vi "WriteFile.vi"(8 "error in (no error)":errorcluster, 11 "Excel refnum":T1) -> (0 "error out":errorcluster, 3 "Excel refnum out":T1)   [LabVIEW 2020, in "NI_ExcelFile.lvlib"]
doc: "Writes data that you logged with the WriteData VI to the specified .xlsx file. After you finish the writing operation, use the Destroy VI to close the reference of the .xlsx file and to delete temporary files.\n \nExcel refnum: Specifies a reference to the .xlsx file on which to perform the operation. Use the Create VI to create or open the refnum.\n\nerror in: describes error conditions that occur before this node runs. This input provides standard error in functionality.\n\nExcel refnum out: Returns a Microsoft Excel file reference to the .xlsx file on which you performed the operation.\n\nerror out: contains error information. This output provides standard error out functionality."
uses:
  <vilib>/express/express shared/NI_ExcelFile/NI_ExcelFile.lvlib
  <vilib>/express/express shared/NI_ExcelFile/Ctrls/ExcelRefnum.ctl
  <vilib>/express/express shared/NI_ExcelFile/Ctrls/MainData.ctl
  <vilib>/express/express shared/NI_ExcelFile/Ctrls/StreamMode.ctl
  <vilib>/express/express shared/NI_ExcelFile/Ctrls/TimeColumnMode.ctl
  <vilib>/express/express shared/NI_ExcelFile/Ctrls/FileAttribute.ctl
  <vilib>/express/express shared/NI_ExcelFile/Ctrls/Columns.ctl
  <vilib>/express/express shared/NI_ExcelFile/Ctrls/ColumnInfo.ctl
  <vilib>/express/express shared/NI_ExcelFile/Ctrls/DataType.ctl
  <vilib>/express/express shared/NI_ExcelFile/Ctrls/wd_recordInfo.ctl
  <vilib>/express/express shared/NI_ExcelFile/Ctrls/disk_TemplateFile.ctl
  <vilib>/express/express shared/NI_ExcelFile/Ctrls/meta_file.ctl
  <vilib>/express/express shared/NI_ExcelFile/Ctrls/meta_Block.ctl
  <vilib>/express/express shared/NI_ExcelFile/Ctrls/meta_BlockType.ctl
  <vilib>/express/express shared/NI_ExcelFile/Ctrls/meta_FileInfo.ctl
  <vilib>/express/express shared/NI_ExcelFile/Ctrls/meta_FileInfo_2013.ctl
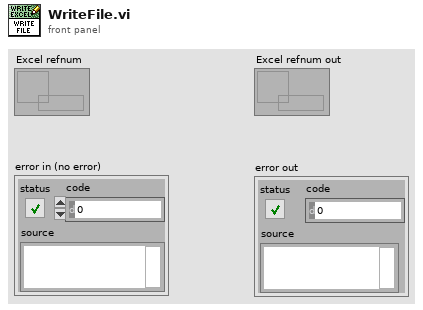
[diagram p1: front panel]
types:
  T1 = typedef "NI_ExcelFile.lvlib/ExcelRefnum.ctl" = refnum<data-value>
  T2 = typedef "NI_ExcelFile.lvlib/meta_FileInfo_2013.ctl" = cluster{"NextPosition":i64, "NextRow":i32, "FileAttribute ":T3}
  T3 = typedef "NI_ExcelFile.lvlib/FileAttribute.ctl" = cluster{"Creator":string, "Title":string, "SheetName":string}
  T4 = typedef "NI_ExcelFile.lvlib/meta_FileInfo.ctl" = cluster{"meta_FileInfo_2013":T2}
  T5 = typedef "NI_ExcelFile.lvlib/MainData.ctl" = cluster{"TargetFile":path, "StreamMode":T6, "Append?":bool, "ChunkSize":u64, "TimeColumnMode":T7, "TimestampFormat":string, "AbsoluteTime?":bool, "FileAttribute ":T3, "Column":T8, "FileRef":refnum<k1>, "MemoryRef":refnum<data-value>[], "RecordInfo":T11[], " ChannelPreviousInfo":u32[], "ChannelFirstRecord":u32[], "PredefinedFormattedValueLength":i64, "DiskTemplate":T12}
  T6 = typedef "NI_ExcelFile.lvlib/StreamMode.ctl" = enum16{"File", "Memory"}
  T7 = typedef "NI_ExcelFile.lvlib/TimeColumnMode.ctl" = enum16{"Empty", "OnePerCh", "One"}
  T8 = typedef "NI_ExcelFile.lvlib/Columns.ctl" = T9[]
  T9 = typedef "NI_ExcelFile.lvlib/ColumnInfo.ctl" = cluster{"Header":string, "Format":string, "DataType":T10, "Length":u64}
  T10 = typedef "NI_ExcelFile.lvlib/DataType.ctl" = enum16{"DDT", "WFM", "Array of STR", "Array of DBL", "Array of I8", "Array of I16", "Array of I32", "Array of I64", "Array of SGL", "Array of U8", "Array of U16", "Array of U32", "Array of U64", "Array of Time"}
  T11 = typedef "NI_ExcelFile.lvlib/wd_recordInfo.ctl" = cluster{"ChannelIndex":u32, "StartIndex":u64, "Length":u64, "Previous":i32, "Next":i32}
  T12 = typedef "NI_ExcelFile.lvlib/disk_TemplateFile.ctl" = cluster{"XMLRef":refnum<file>[], "ZipPath":path, "MetaFile":T13, "TempFolder":path}
  T13 = typedef "NI_ExcelFile.lvlib/meta_file.ctl" = cluster{"Ref":refnum<file>, "NextRow":i32, "NextPosition":i64, "Block":T14[]}
  T14 = typedef "NI_ExcelFile.lvlib/meta_Block.ctl" = cluster{"Version":u16, "Type":T15, "Length":i32, "Data":string}
  T15 = typedef "NI_ExcelFile.lvlib/meta_BlockType.ctl" = enum16{"NITag", "File", "Column"}
  T16 = typedef "NI_ExcelFile.lvlib/fmt_formatBuffer.ctl" = cluster{"FormatBuffer":u8[], "BufferIndices":i32[], "CellFormatBuffer":u8[], "FormatBufferWidth":i32, "FormattedDataLength":i32, "MaxRow":i32, "StartRow":i32, "TimeColumnMode":T7, "StartTime":timestamp, "Columns":T8, "ActualLength":i32}
  T17 = typedef "NI_ExcelFile.lvlib/data_AllTypeData.ctl" = cluster{"DataType":T10, "DBL":dbl[], "WFM":waveform(dbl), "STR":string[], "Time":timestamp[], "I8":i8[], "I16":i16[], "I32":i32[], "I64":i64[], "SGL":sgl[], "U8":u8[], "U16":u16[], "U32":u32[], "U64":u64[]}
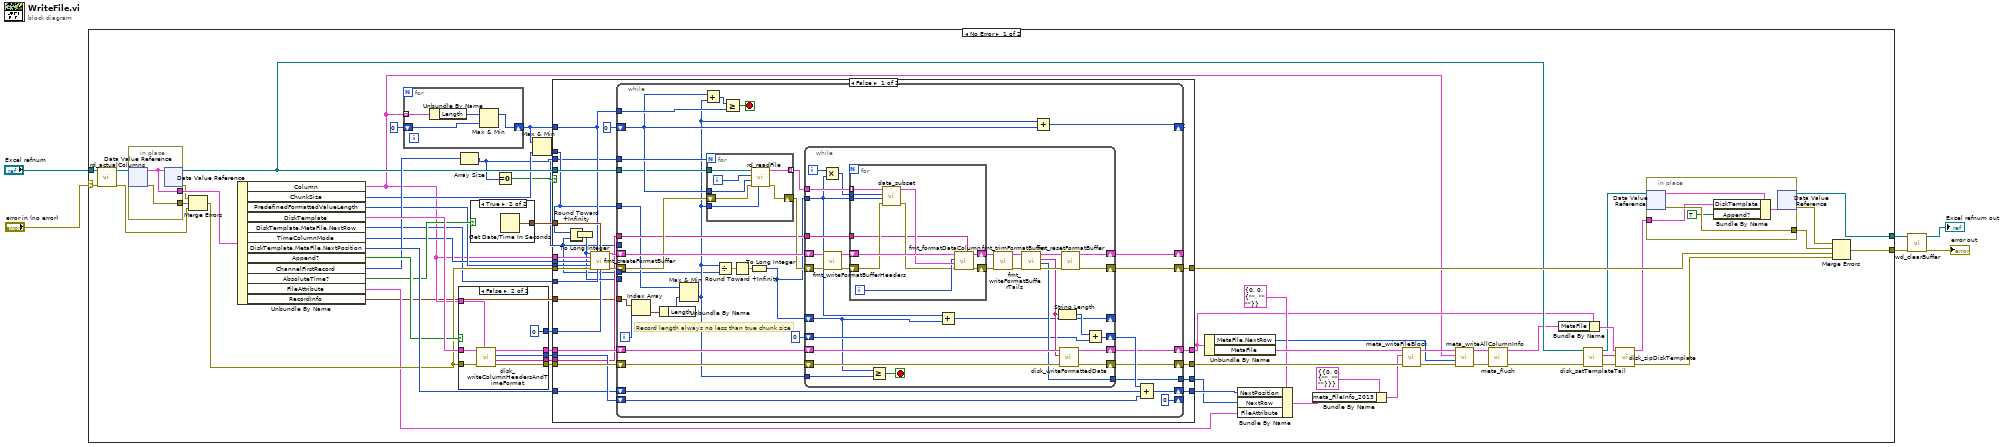
[diagram p0: block diagram]
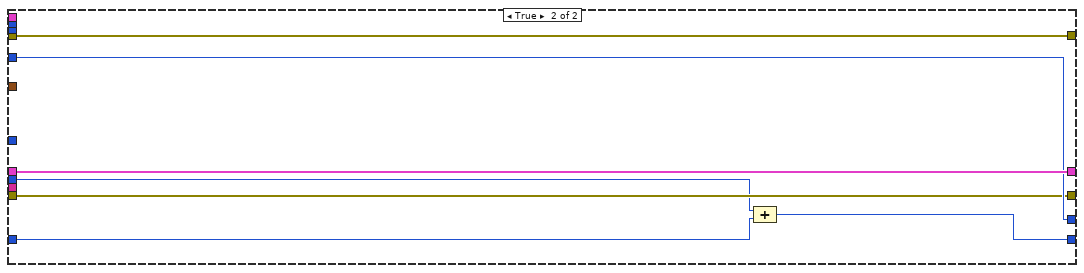
[diagram p2: hidden frame]
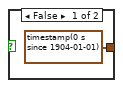
[diagram p3: hidden frame]
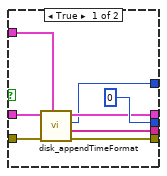
[diagram p4: hidden frame]
diagram:
  n1 = case shown="No Error" "error in (no error)" {
    selector: "error in (no error)" -> [w46 w214]
    tunnel: "Excel refnum" -> [w47 w213]
    tunnel: [w27 w214] -> w2
    tunnel: [w28 w213] -> w4
    frame No Error {
      n2 = call <vilib>:"rd_actualColumns.vi"("error in (no error)"=w46, "Excel refnum"=w47) -> ("errorout"=w45:errorcluster, "Excel refnum out"=w44:T1)  [unwired: 8 in]
      n3 = in-place {
        in-place-border: [w212] -> w60
        in-place-border: [w211] -> w58
        n4 = in-place-dvr #1(w44) -> (w212:T5, w211:errorcluster)
        n5 = in-place-dvr #1(w212) -> (w32:T1, w59:errorcluster)
      }
      n6 = Merge Errors(w59, w58, w45) -> (w43:errorcluster)
      n7 = Unbundle By Name(w60) -> ("Column"=w9:T8, "ChunkSize"=w22:u64, "PredefinedFormattedValueLength"=w26:i64, "DiskTemplate"=w64:T12, "DiskTemplate.MetaFile.NextRow"=w24:i32, "TimeColumnMode"=w25:T7, "DiskTemplate.MetaFile.NextPosition"=w53:i64, "Append?"=w50:bool, "ChannelFirstRecord"=w42:u32[], "AbsoluteTime?"=w41:bool, "FileAttribute"=w13:T3, "RecordInfo"=w7:T11[])
      n8 = for {
        tunnel: w9 -> [w189] mode=indexing
        shift-right: [w188] -> w23
        shift-left: u64 0 ("Column Length") -> [w186]
        n9 = Unbundle By Name(w189) -> ("Length"=w187:u64)
        n10 = Max & Min(x=w187, y=w186) -> (max(x,y)=w188:u64)  [unwired: 1 out]
      }
      n11 = case shown="False" w50 {
        tunnel: w64 -> [w192 w205]
        tunnel: [w191 w204] -> w63
        tunnel: [w195 w203] -> w62
        tunnel: [0 ("formatted header length") w202] -> w61
        tunnel: w43 -> [w196 w199]
        tunnel: [w194 w201] -> w48
        tunnel: w9 -> [w193 w200]
        tunnel: [w190 0 ("max existed styles")] -> w8
        frame True {
          n12 = call <vilib>:"disk_appendTimeFormat.vi"("columns"=w193, "error in (no error)"=w196, "DiskTemplate"=w192) -> ("error out"=w195:errorcluster, "styles map"=w194:string[], "max existed styles"=w190:i32, "DiskTemplate out"=w191:T12)  [unwired: 5 in]
        }
        frame False {
          n13 = call <vilib>:"disk_writeColumnHeadersAndTimeFormat.vi"("column"=w200, "error in"=w199, "DiskTemplate in"=w205) -> ("error out"=w203:errorcluster, "styles map"=w201:string[], "formatted header length"=w202:i32, "DiskTemplate out"=w204:T12)  [unwired: 5 in]
        }
      }
      n14 = Array Size(array=w42) -> (size(s)=w12:i32)
      n15 = case shown="True" w41 {
        tunnel: [timestamp(0 s since 1904-01-01) ("start time") w185] -> w40
        frame False {
        }
        frame True {
          n16 = Get Date/Time In Seconds() -> (seconds since 1Jan1904=w185:timestamp)
        }
      }
      n17 = Equal To 0?(x=w12) -> (x = 0?=w11:bool)
      n18 = Max & Min(x=w23, y=w22) -> (min(x,y)=w14:u64)  [unwired: 1 out]
      n19 = case shown="False" w11 {
        tunnel: [w93 w180] -> w65
        tunnel: w63 -> [w89 w183]
        tunnel: w62 -> [w88 w181]
        tunnel: w61 -> [w87 w179]
        tunnel: w53 -> [w86 w178]
        tunnel: [w84 w181] -> w52
        tunnel: w48 -> [w83 _]
        tunnel: w43 -> [w82 w180]
        tunnel: w40 -> [w81 _]
        tunnel: [w80 w177] -> w34
        tunnel: [w79 w182] -> w33
        tunnel: w32 -> [w78 _]
        tunnel: w26 -> [w77 _]
        tunnel: w25 -> [w76 _]
        tunnel: w24 -> [w75 w182]
        tunnel: w23 -> [w74 _]
        tunnel: w14 -> [w73 _]
        tunnel: w9 -> [w72 _]
        tunnel: w12 -> [w66 _]
        tunnel: [w85 w183] -> w10
        tunnel: w8 -> [w68 _]
        tunnel: w7 -> [w67 _]
        frame False {
          n20 = Divide(x=w73, y=w66) -> (x/y=w70:dbl)
          n21 = Round Toward +Infinity(x=w70) -> (ceil(x): smallest int >= x=w69:dbl)
          n22 = To Long Integer(number=w69) -> (32bit integer=w71:i32)
          n23 = call <vilib>:"fmt_createFormatBuffer.vi"("rows"=w71, "max rows"=w74, "start time"=w81, "columns"=w72, "time column mode"=w76, "predifed formatted value length"=w77, "error in (no error)"=w82, "start row"=w75, "max styles"=w68) -> ("Format buffers out"=w90:T16, "error out"=w91:errorcluster)  [unwired: 5 in]
          n24 = while {
            tunnel: w66 -> [w128]
            tunnel: w74 -> [w127]
            shift-right: [w124] -> w93
            shift-left: w91 -> [w108]
            shift-right: [w114] -> w85
            shift-left: w89 -> [w117]
            shift-right: [w123] -> _
            shift-left: u64 0 ("Trunck size") -> [w120]
            shift-right: [w122] -> _
            shift-left: w90 -> [w125]
            tunnel: w73 -> [w100]
            tunnel: w78 -> [w119]
            shift-right: [w115] -> w84
            shift-left: w88 -> [w118]
            shift-right: [w113] -> w80
            shift-left: w86 -> [w112]
            tunnel: [w110] -> w79
            tunnel: w83 -> [w106]
            shift-right: [0 ("formatted header length")] -> _
            shift-left: w87 -> [w111]
            tunnel: w66 -> [_]
            tunnel: w71 -> [_]
            tunnel: w67 -> [w103]
            tunnel: w66 -> [w96]
            i -> [w102]
            stop <- w126 stop-if-true
            # "Record length always no less than true chunk size"
            n25 = Index Array(array=w103, index=w102) -> (element=w101:T11)
            n26 = Unbundle By Name(w101) -> ("Length"=w94:u64)
            n27 = Max & Min(x=w100, y=w94) -> (min(x,y)=w97:u64)  [unwired: 1 out]
            n28 = Add(x=w120, y=w97) -> (x+y=w121:u64)
            n29 = for {
              N: w128 -> [_]
              tunnel: w97 -> [w175]
              tunnel: w120 -> [w176]
              tunnel: w119 -> [w174]
              shift-right: [w171] -> w107
              shift-left: w108 -> [w172]
              tunnel: [w170] -> w105 mode=indexing
              i -> [w173]
              n30 = call <vilib>:"rd_readFile.vi"("length"=w175, "error in (no error)"=w172, "start index"=w176, "channel index"=w173, "Excel refumn"=w174) -> ("error out"=w171:errorcluster, "data_AllTypeData"=w170:T17)  [unwired: 5 in]
            }
            n31 = Divide(x=w97, y=w96) -> (x/y=w99:dbl)
            n32 = Greater Or Equal?(x=w121, y=w127) -> (x >= y?=w126:bool)
            n33 = Round Toward +Infinity(x=w99) -> (ceil(x): smallest int >= x=w98:dbl)
            n34 = To Long Integer(number=w98) -> (32bit integer=w95:i32)
            n35 = while {
              tunnel: [w145] -> w110
              shift-right: [w152] -> w122
              shift-left: w125 -> [w158]
              shift-right: [w153] -> w124
              shift-left: w107 -> [w154]
              shift-right: [w147] -> w115
              shift-left: w118 -> [w150]
              shift-right: [w146] -> w114
              shift-left: w117 -> [w149]
              shift-right: [w140] -> w116
              shift-left: 0 -> [w139]
              tunnel: w105 -> [w137]
              tunnel: w106 -> [w136]
              tunnel: w95 -> [w130]
              shift-right: [w133] -> _
              shift-left: w95 -> [w129]
              tunnel: w97 -> [w132]
              i -> [w135]
              stop <- w131 stop-if-true
              n36 = Multiply(x=w135, y=w130) -> (x*y=w134:i32)
              n37 = call <vilib>:"fmt_writeFormatBufferHeaders.vi"("error in (no error)"=w154, "Format buffers in"=w158) -> ("error out"=w141:errorcluster, "Format buffers out"=w142:T16)  [unwired: 8 in]
              n38 = for {
                shift-right: [w168] -> w143
                shift-left: w142 -> [w167]
                shift-right: [w169] -> w144
                shift-left: w141 -> [w162]
                tunnel: w137 -> [w166] mode=indexing
                tunnel: w136 -> [w161]
                tunnel: w134 -> [w160]
                tunnel: w130 -> [w159]
                i -> [w164]
                n39 = call <vilib>:"data_subset.vi"("error in (no error)"=w162, "length"=w159, "index"=w160, "data"=w166) -> ("error out"=w163:errorcluster, "data subset"=w165:T17)  [unwired: 6 in]
                n40 = call <vilib>:"fmt_formatDataColumn.vi"("styles map"=w161, "error in (no error)"=w163, "data"=w165, "channel index"=w164, "Format buffers in"=w167) -> ("error out"=w169:errorcluster, "Format buffers out"=w168:T16)  [unwired: 5 in]
              }
              n41 = Greater Or Equal?(x=w129, y=w132) -> (x >= y?=w131:bool)
              n42 = Add(x=w130, y=w129) -> (x+y=w133:i32)
              n43 = call <vilib>:"fmt_writeFormatBufferTails.vi"("error in (no error)"=w144, "Format buffers in"=w143) -> ("error out"=w156:errorcluster, "Format buffers out"=w157:T16)  [unwired: 8 in]
              n44 = call <vilib>:"fmt_trimFormatBuffer.vi"("error in (no error)"=w156, "format buffers in"=w157) -> ("error out"=w151:errorcluster, "max row"=w145:i32, "xml"=w148:string, "format buffers out"=w155:T16)  [unwired: 6 in]
              n45 = String Length(string=w148) -> (length=w138:i32)
              n46 = call <vilib>:"disk_writeFormattedData.vi"("error in"=w150, "xml"=w148, "DiskTemplate in"=w149) -> ("error out"=w147:errorcluster, "DiskTemplate out"=w146:T12)  [unwired: 7 in]
              n47 = call <vilib>:"fmt_resetFormatBuffer.vi"("error in (no error)"=w151, "Format buffers in"=w155) -> ("error out"=w153:errorcluster, "Format buffers out"=w152:T16)  [unwired: 8 in]
              n48 = Add(x=w138, y=w139) -> (x+y=w140:i32)
            }
            n49 = Add(x=w97, y=w120) -> (x+y=w123:u64)
            n50 = Compound Arithmetic op=ADD(w116, w112, w111) -> (w113:i64)
          }
        }
        frame True {
          n51 = Compound Arithmetic op=ADD(w179, w178) -> (w177:i64)
        }
      }
      n52 = Unbundle By Name(w10) -> ("MetaFile.NextRow"=w15:i32, "MetaFile"=w39:T13)
      n53 = Bundle By Name(cluster=T2 {"NextPosition"=0, "NextRow"=0, "FileAttribute "={"Creator"="", "Title"="", "SheetName"=""}} ("meta_FileInfo_2013"), "NextPosition"=w34, "NextRow"=w33, "FileAttribute"=w13) -> (w36:T2)
      n54 = Bundle By Name(cluster=T4 {"meta_FileInfo_2013"={"NextPosition"=0, "NextRow"=0, "FileAttribute "={"Creator"="", "Title"="", "SheetName"=""}}} ("meta_FileInfo"), "meta_FileInfo_2013"=w36) -> (w37:T4)
      n55 = call <vilib>:"meta_writeFileBlock.vi"("error in (no error)"=w52, "meta_FileInfo"=w37, "meta file in"=w39) -> ("error out"=w21:errorcluster, "meta file out"=w20:T13)  [unwired: 7 in]
      n56 = call <vilib>:"meta_writeAllColumnInfo.vi"("error in (no error)"=w21, "start row"=w15, "Column"=w9, "meta file in"=w20) -> ("error out"=w19:errorcluster, "meta file out"=w16:T13)  [unwired: 6 in]
      n57 = call <vilib>:"meta_flush.vi"("error in (no error)"=w19, "meta file in"=w16) -> ("error out"=w18:errorcluster, "meta file out"=w17:T13)  [unwired: 8 in]
      n58 = Bundle By Name(cluster=w10, "MetaFile"=w17) -> (w51:T12)
      n59 = call <vilib>:"disk_setTemplateTail.vi"("error in (no error)"=w18, "Excel refnum"=w32) -> ("error out"=w31:errorcluster, "template tail"=w30:string[], "Excel refnum out"=w29:T1)  [unwired: 7 in]
      n60 = call <vilib>:"disk_zipDiskTemplate.vi"("error in (no error)"=w31, "template tail"=w30, "DiskTemplate in"=w51) -> ("error out"=w54:errorcluster, "DiskTemplate out"=w55:T12)  [unwired: 7 in]
      n61 = in-place {
        in-place-border: [w210] -> w56
        in-place-border: w55 -> [w207]
        n62 = in-place-dvr #2(w29) -> (w209:T5, w210:errorcluster)
        n63 = Bundle By Name(cluster=w209, "DiskTemplate"=w207, "Append?"=TRUE ("Append")) -> (w208:T5)
        n64 = in-place-dvr #2(w208) -> (w28:T1, w57:errorcluster)
      }
      n65 = Merge Errors(w57, w56, w65, w54) -> (w27:errorcluster)
    }
    frame Error {
    }
  }
  n66 = call <vilib>:"wd_clearBuffer.vi"("error in (no error)"=w2, "Excel refnum in"=w4) -> ("error out"=→"error out":errorcluster, "Excel refnum out"=→"Excel refnum out":T1)  [unwired: 8 in]
